vi "WaveformArrayMinusRingTime.vi"(10 "RT Index":dbl, 11 "Pre-cut Waveforms":waveform(dbl)[](array[waveform])) -> (3 "Post-cut Waveforms":waveform(dbl)[](array[waveform]))   [LabVIEW 2019]
panel:
  out "Waveform Graph 2":waveform(dbl)[](graph)
  out "Waveform Graph":waveform(dbl)[](graph)
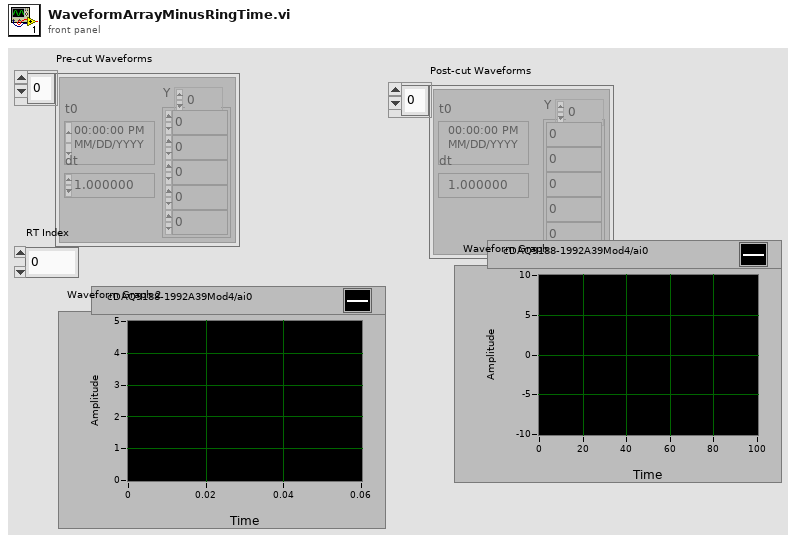
[diagram p1: front panel]
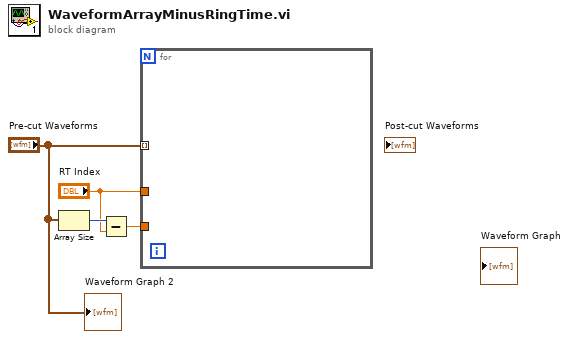
[diagram p0: block diagram]
diagram:
  n1 = Array Size(array="Pre-cut Waveforms") -> (size(s)=w4:i32)
  n2 = Subtract(x=w4, y="RT Index") -> (x-y=w2:dbl)
  n3 = for {
    tunnel: "Pre-cut Waveforms" -> [_] mode=indexing
    tunnel: "RT Index" -> [_]
    tunnel: w2 -> [_]
  }
  "Waveform Graph 2" <- "Pre-cut Waveforms"
